vi "ReadEyeFileFast.vi"(0 "new file path":path=path "C:/WINDOWS/DESKTOP/rri.eye", 6 "Header format":u16(ring) items=["Riverside Format", "Ron Linear", "GE Bin"]) -> (8 "Complex output array":csg[][](array[numeric]), 9 "Digitizer (dB)":sgl, 10 "new path out":path, 11 "RF Att":sgl format="%.2f", 13 "2-D data array":sgl[][](array[numeric]), 14 "Header In":T1={"header info"={"Header"="", "Head length"=0}, "A/D info"={"# rf points per line"=0, "# lines per scan"=0, "sample rate MHz"=0, "# A/D bits"=0, "# bytes per A/D"=0, "TGC Flag"=0, "A/D Type"=""}, "Tranducer Info"={"bandwidth"=0.0, "center freq"=0.0, "start freq"=0.0, "ID"=0}, "Scan Info"={"delay"=0.0, "pivot distance"=0.0, "sector scan angle"=0.0, "operator"="", "Scan Mode"="", "location"=""}, "Time/Date Info"={"date"="", "time"=""}, "RF Info"={"RF file name"="", "RF file att"="", "RF cal file name"="", "RF cal file att"=""}, "Patient Info"={"ID"="", "extended ID"="", "age"=0, "sex"="", "previously\nscanned"="", "PSA"=0.0, "LOS"=1, "Ethnicty 2"=3, "Race"=3}, "Tissue Type"={"organ"=0, "disease type"=0, "disease location"=0, "IQ_pts"=0, "RcvBuffer"=0, "RcvFrame"=0, "IQBuff"=0, "IQFrame"=0, "IQPage"=0}, "Votage scaling"={"Digitizer (dB)"=0.0, "Gain (dB)"=0.0, "Atten (dB)"=0.0}, "Comment"="", "Misc Info"={"avg num"=0, "c speed"=0, "Div By or SF zones"=0, "XMIT CHS"=0, "RCV CHS"=0, "Xmit angle"=0.0}, "Therapy Parameters"={"Theraputic Freq (MHz)"=0.0, "Time on (s)"=0.0, "Therapy amplitude (mV)"=0.0, "Lines Before"=0, "Lines After"=0}, "Scan Settings"={"Energy (uJ or V)"=0, "Damp (Ohm) or Fc"=0, "HP Filt (KHz)"=0, "LP Filt (MHz)"=0, "Gain (db)"=0, "prf (kHz)"=0.0, "Distance between\nscan lines (um)"=0, "Distance between\nscan planes (um)"=0, "Scan line gap (um)"=0.0, "Scan plane gap (um)"=0.0}, "Compression Parameters"={"F1 (MHz)"=0.0, "F2 (MHz)"=0.0, "% taper"=0.0, "duration"=0.0}, "Patient Info Xtra"={"First Name"="", "Last Name"="", "Notes"=""}, "ROI Box"=[0, 0, 0, 0]} {"Compression Parameters"."% taper" min=50 max=1000 format="%.2f"; "Compression Parameters"."F2 (MHz)" format="%.3f"; "Compression Parameters"."F1 (MHz)" format="%.3f"; "Scan Settings"."prf (kHz)" format="%.2f"; "Therapy Parameters"."Therapy amplitude (mV)" min=50 max=1000 format="%.2f"; "Therapy Parameters"."Time on (s)" format="%.3f"; "Therapy Parameters"."Theraputic Freq (MHz)" format="%.3f"; "Patient Info"."Race" items=["Am Ind or Alaska", "Asian", "Hawaiian, Pac Isl", "Black or Afr Amer", "White", "more than one race", "unknown"]; "Patient Info"."Ethnicty 2" items=["Hispanic", "Non-Hispanic", "unknown"]; "Patient Info"."LOS" items=["1", "2", "3", "4", "5"]; "Patient Info"."PSA" format="%.1f"; "Scan Info"."delay" format="%.2f"; "Scan Info"."pivot distance" format="%.2f"; "Scan Info"."sector scan angle" format="%.2f"; "Tranducer Info"."bandwidth" format="%.2f"; "Tranducer Info"."center freq" format="%.2f"; "Tranducer Info"."start freq" format="%.2f"})   [LabVIEW 2022 SP3]
uses:
  Header.ctl
panel:
  out "error out":errorcluster
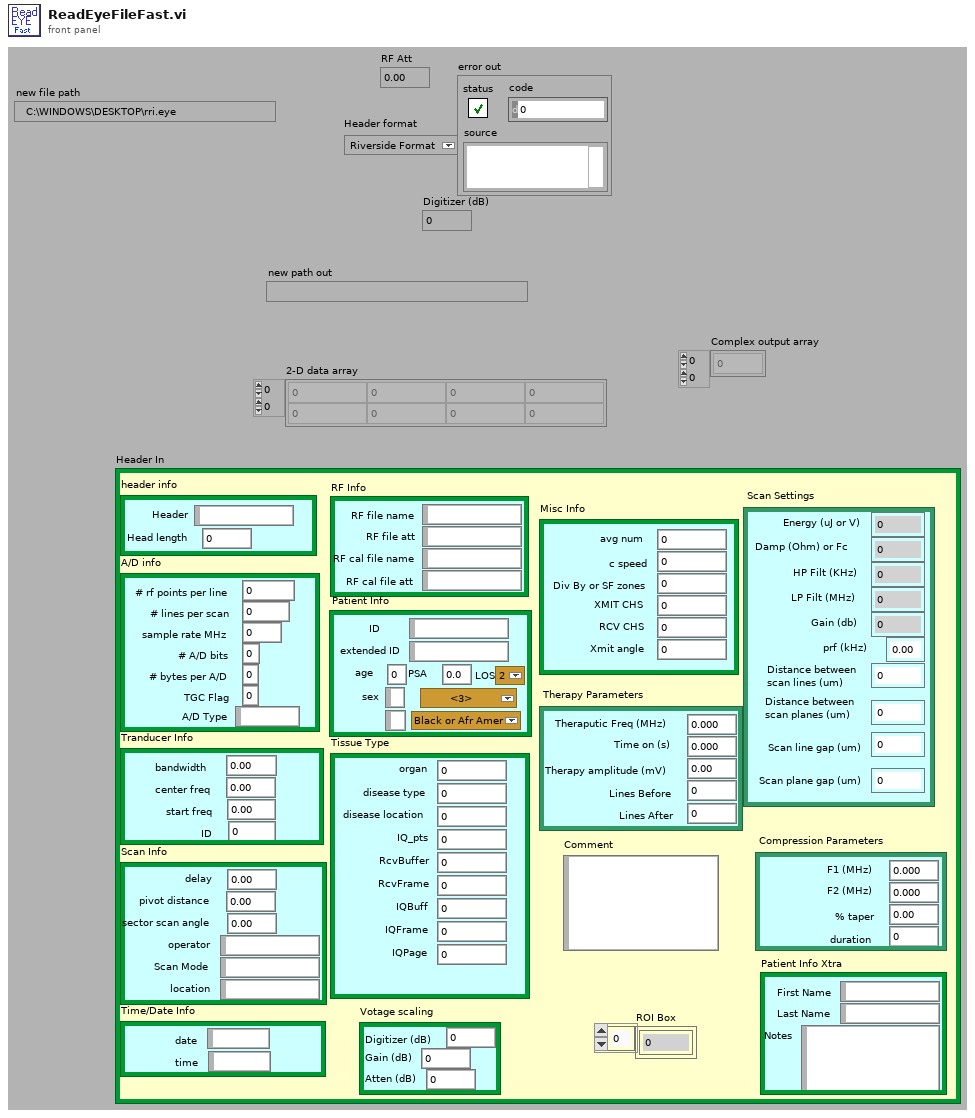
[diagram p1: front panel]
types:
  T1 = typedef "Header.ctl" = cluster{"header info":cluster{"Header":string, "Head length":i16}, "A/D info":cluster{"# rf points per line":u16, "# lines per scan":u16, "sample rate MHz":u16, "# A/D bits":i16, "# bytes per A/D":u16, "TGC Flag":u16, "A/D Type":string}, "Tranducer Info":cluster{"bandwidth":sgl, "center freq":sgl, "start freq":sgl, "ID":i32}, "Scan Info":cluster{"delay":sgl, "pivot distance":sgl, "sector scan angle":sgl, "operator":string, "Scan Mode":string, "location":string}, "Time/Date Info":cluster{"date":string, "time":string}, "RF Info":cluster{"RF file name":string, "RF file att":string, "RF cal file name":string, "RF cal file att":string}, "Patient Info":cluster{"ID":string, "extended ID":string, "age":u16, "sex":string, "previously\nscanned":string, "PSA":sgl, "LOS":u8, "Ethnicty 2":u8, "Race":u8}, "Tissue Type":cluster{"organ":i16, "disease type":i16, "disease location":i16, "IQ_pts":u16, "RcvBuffer":u8, "RcvFrame":u16, "IQBuff":u8, "IQFrame":u16, "IQPage":u8}, "Votage scaling":cluster{"Digitizer (dB)":sgl, "Gain (dB)":sgl, "Atten (dB)":sgl}, "Comment":string, "Misc Info":cluster{"avg num":u16, "c speed":i16, "Div By or SF zones":i16, "XMIT CHS":u8, "RCV CHS":u8, "Xmit angle":sgl}, "Therapy Parameters":cluster{"Theraputic Freq (MHz)":sgl, "Time on (s)":sgl, "Therapy amplitude (mV)":sgl, "Lines Before":u16, "Lines After":u16}, "Scan Settings":cluster{"Energy (uJ or V)":u8, "Damp (Ohm) or Fc":u8, "HP Filt (KHz)":u8, "LP Filt (MHz)":u8, "Gain (db)":u8, "prf (kHz)":sgl, "Distance between\nscan lines (um)":u16, "Distance between\nscan planes (um)":u16, "Scan line gap (um)":sgl, "Scan plane gap (um)":sgl}, "Compression Parameters":cluster{"F1 (MHz)":sgl, "F2 (MHz)":sgl, "% taper":sgl, "duration":sgl}, "Patient Info Xtra":cluster{"First Name":string, "Last Name":string, "Notes":string}, "ROI Box":u16[]}
  T2 = enum16{"big-endian, network order", "native, host order", "little-endian"}
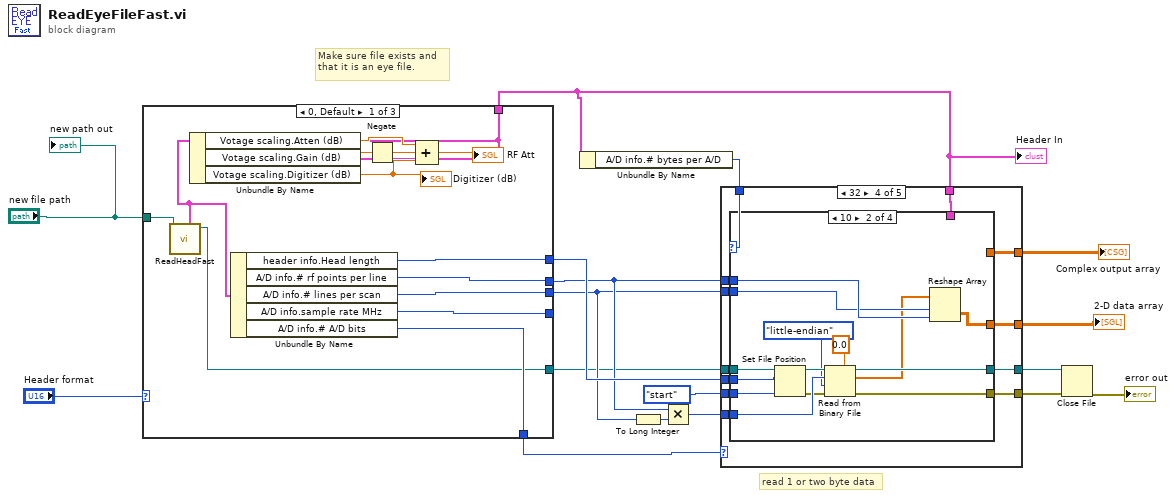
[diagram p0: block diagram]
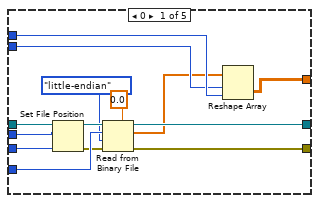
[diagram p2: hidden frame]
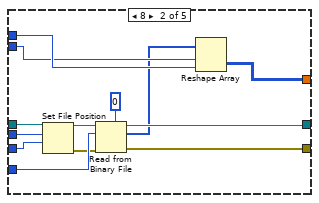
[diagram p3: hidden frame]
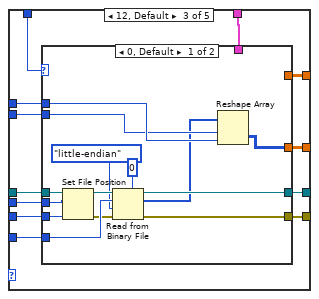
[diagram p4: hidden frame]
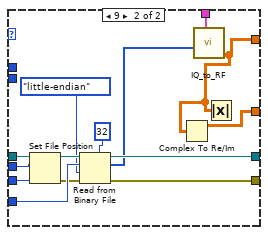
[diagram p5: hidden frame]
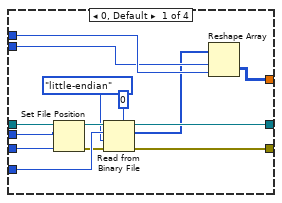
[diagram p6: hidden frame]
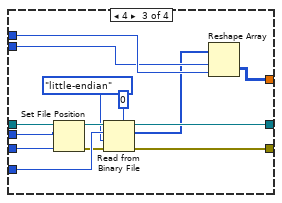
[diagram p7: hidden frame]
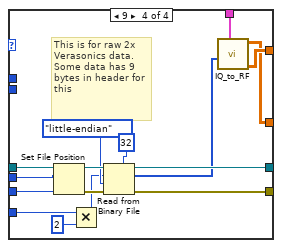
[diagram p8: hidden frame]
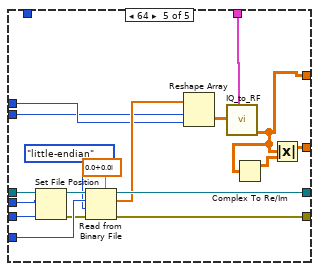
[diagram p9: hidden frame]
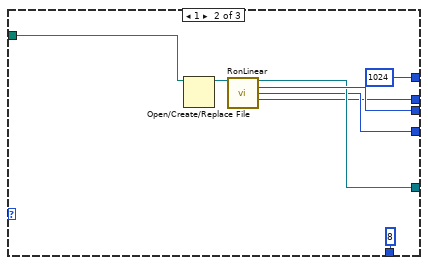
[diagram p10: hidden frame]
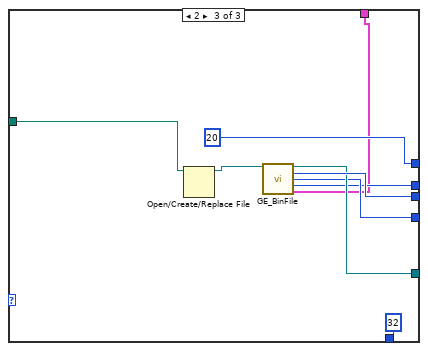
[diagram p11: hidden frame]
diagram:
  # "Make sure file exists and that it is an eye file."
  # "read 1 or two byte data"
  n1 = case shown="0, Default" "Header format" {
    tunnel: [w26 w35 w44] -> _
    tunnel: [w28 w33 w42] -> w7
    tunnel: [w27 w38 w47] -> w6
    tunnel: [w19 w37 w46] -> w2
    tunnel: [w29 i16 1024 i16 20] -> w12
    tunnel: [w25 8 32] -> w8
    tunnel: "new file path" -> [w30 w31 w40]
    tunnel: [w18 _ w39] -> w4
    frame 0, Default {
      n2 = call "ReadHeadFast.vi"("new file path"=w30) -> ("refnum out"=w19:refnum<file>, "Header In"=w18:T1)  [unwired: 7 in, 2 out]
      n3 = Unbundle By Name(w18) -> ("Votage scaling.Atten (dB)"=w20:sgl, "Votage scaling.Gain (dB)"=w23:sgl, "Votage scaling.Digitizer (dB)"=w24:sgl)
      "Digitizer (dB)" <- w24
      n4 = Unbundle By Name(w18) -> ("header info.Head length"=w29:i16, "A/D info.# rf points per line"=w28:u16, "A/D info.# lines per scan"=w27:u16, "A/D info.sample rate MHz"=w26:u16, "A/D info.# A/D bits"=w25:i16)
      n5 = Negate(x=w23) -> (-x=w21:sgl)
      n6 = Compound Arithmetic op=ADD(w20, w21, w24) -> (→"RF Att":sgl)
    }
    frame 1 {
      n7 = Open/Create/Replace File(file path (use dialog)=w31) -> (refnum out=w32:refnum<file>)  [unwired: 5 in, 2 out]
      n8 = call "RonLinear.vi"("refnum"=w32) -> ("refnum out"=w37:refnum<file>, "# lines per scan"=w38:i32, "sample rate"=w35:u16, "# rf points per line"=w33:u16)  [unwired: 11 out]
    }
    frame 2 {
      n9 = Open/Create/Replace File(file path (use dialog)=w40) -> (refnum out=w41:refnum<file>)  [unwired: 5 in, 2 out]
      n10 = call "GE_BinFile.vi"("refnum"=w41) -> ("refnum out"=w46:refnum<file>, "# lines per scan"=w47:i32, "sample rate"=w44:u16, "# rf points per line"=w42:u16, "Header In"=w39:T1)  [unwired: 9 in, 1 out]
    }
  }
  "Header In" <- w4
  n11 = Unbundle By Name(w4) -> ("A/D info.# bytes per A/D"=w5:u16)
  n12 = To Long Integer(number=w6) -> (32bit integer=w15:i32)
  n13 = Multiply(x=w7, y=w15) -> (x*y=w16:i32)
  n14 = case shown="32" w8 {
    tunnel: enum16{"start", "end", "current"}."start" ("pos mode (0:2)") -> [w58 w73 w84 w124 w198]
    tunnel: [w48 w62 w78 w118 w185] -> w3
    tunnel: w16 -> [w59 w72 w85 w125 w199]
    tunnel: w2 -> [w61 w71 w86 w126 w201]
    tunnel: w12 -> [w54 w70 w82 w122 w194]
    tunnel: [w57 w69 w83 w123 w197] -> w13
    tunnel: [w52 w66 w81 w121 w192] -> w11
    tunnel: w7 -> [w51 w65 w80 w120 w190]
    tunnel: w6 -> [w50 w64 w79 w119 w189]
    tunnel: w4 -> [_ _ w76 w116 w188]
    tunnel: w5 -> [_ _ w77 w117 _]
    tunnel: [_ _ w75 w115 w186] -> w1
    frame 0 {
      n15 = Set File Position(offset (in bytes) (0)=w54, refnum=w61, from (0:start)=w58) -> (refnum out=w56:refnum<file>, error out=w55:errorcluster)  [unwired: 1 in]
      n16 = Read from Binary File(5:sgl 0.0, 8:w55, 9:T2."little-endian" ("byte order (0:big-endian, network order)"), 10:w59, 11:w56) -> (0:w52:errorcluster, 2:w49:sgl[], 3:w57:refnum<file>)  [unwired: 2 out]
      n17 = Reshape Array(w49, w50, w51) -> (w48:sgl[][])
    }
    frame 8 {
      n18 = Set File Position(offset (in bytes) (0)=w70, refnum=w71, from (0:start)=w73) -> (refnum out=w68:refnum<file>, error out=w67:errorcluster)  [unwired: 1 in]
      n19 = Read from Binary File(5:i8 0, 8:w67, 10:w72, 11:w68) -> (0:w66:errorcluster, 2:w63:i8[], 3:w69:refnum<file>)  [unwired: 3 out]
      n20 = Reshape Array(w63, w64, w65) -> (w62:i8[][])
    }
    frame 12, Default {
      n21 = case shown="0, Default" w77 {
        tunnel: w86 -> [w100 w114]
        tunnel: w85 -> [w98 w112]
        tunnel: w84 -> [w97 w111]
        tunnel: [w96 w110] -> w83
        tunnel: w82 -> [w93 w107]
        tunnel: [w91 w105] -> w81
        tunnel: w80 -> [w90 _]
        tunnel: w79 -> [w89 _]
        tunnel: [w87 w101] -> w78
        tunnel: w76 -> [_ w104]
        tunnel: [_ w102] -> w75
        frame 0, Default {
          n22 = Set File Position(offset (in bytes) (0)=w93, refnum=w100, from (0:start)=w97) -> (refnum out=w95:refnum<file>, error out=w94:errorcluster)  [unwired: 1 in]
          n23 = Read from Binary File(5:i16 0, 8:w94, 9:T2."little-endian" ("byte order (0:big-endian, network order)"), 10:w98, 11:w95) -> (0:w91:errorcluster, 2:w88:i16[], 3:w96:refnum<file>)  [unwired: 2 out]
          n24 = Reshape Array(w88, w89, w90) -> (w87:i16[][])
        }
        frame 9 {
          n25 = Set File Position(offset (in bytes) (0)=w107, refnum=w114, from (0:start)=w111) -> (refnum out=w109:refnum<file>, error out=w108:errorcluster)  [unwired: 1 in]
          n26 = Read from Binary File(5:32, 8:w108, 9:T2."little-endian" ("byte order (0:big-endian, network order)"), 10:w112, 11:w109) -> (0:w105:errorcluster, 2:w103:i32[], 3:w110:refnum<file>)  [unwired: 2 out]
          n27 = call "IQ_to_RF.vi"("Header In"=w104, "IQ Array In"=w103) -> ("Z Out"=w102:csg[][])  [unwired: 8 in, 1 out]
          n28 = Complex To Re/Im(x + iy=w102) -> (x=w101:sgl[][])  [unwired: 1 out]
          n29 = Absolute Value(x=w102) -> ()  [unwired: 1 out]
        }
      }
    }
    frame 32 {
      n30 = case shown="10" w117 {
        tunnel: w126 -> [w140 w154 w168 w184]
        tunnel: w125 -> [w138 w152 w166 w173]
        tunnel: w124 -> [w137 w151 w165 w182]
        tunnel: [w136 w150 w164 w181] -> w123
        tunnel: w122 -> [w133 w147 w161 w178]
        tunnel: [w131 w145 w159 w176] -> w121
        tunnel: w120 -> [w130 w144 w158 _]
        tunnel: w119 -> [w129 w143 w157 _]
        tunnel: [w127 w141 w155 w169] -> w118
        tunnel: w116 -> [_ _ _ w175]
        tunnel: [_ _ _ w170] -> w115
        frame 0, Default {
          n31 = Set File Position(offset (in bytes) (0)=w133, refnum=w140, from (0:start)=w137) -> (refnum out=w135:refnum<file>, error out=w134:errorcluster)  [unwired: 1 in]
          n32 = Read from Binary File(5:0, 8:w134, 9:T2."little-endian" ("byte order (0:big-endian, network order)"), 10:w138, 11:w135) -> (0:w131:errorcluster, 2:w128:i32[], 3:w136:refnum<file>)  [unwired: 2 out]
          n33 = Reshape Array(w128, w129, w130) -> (w127:i32[][])
        }
        frame 10 {
          n34 = Set File Position(offset (in bytes) (0)=w147, refnum=w154, from (0:start)=w151) -> (refnum out=w149:refnum<file>, error out=w148:errorcluster)  [unwired: 1 in]
          n35 = Read from Binary File(5:sgl 0.0, 8:w148, 9:T2."little-endian" ("byte order (0:big-endian, network order)"), 10:w152, 11:w149) -> (0:w145:errorcluster, 2:w142:sgl[], 3:w150:refnum<file>)  [unwired: 2 out]
          n36 = Reshape Array(w142, w143, w144) -> (w141:sgl[][])
        }
        frame 4 {
          n37 = Set File Position(offset (in bytes) (0)=w161, refnum=w168, from (0:start)=w165) -> (refnum out=w163:refnum<file>, error out=w162:errorcluster)  [unwired: 1 in]
          n38 = Read from Binary File(5:0, 8:w162, 9:T2."little-endian" ("byte order (0:big-endian, network order)"), 10:w166, 11:w163) -> (0:w159:errorcluster, 2:w156:i32[], 3:w164:refnum<file>)  [unwired: 2 out]
          n39 = Reshape Array(w156, w157, w158) -> (w155:i32[][])
        }
        frame 9 {
          # "This is for raw 2x\nVerasonics data.\nSome data has 9 bytes in header for this"
          n40 = Set File Position(offset (in bytes) (0)=w178, refnum=w184, from (0:start)=w182) -> (refnum out=w180:refnum<file>, error out=w179:errorcluster)  [unwired: 1 in]
          n41 = Multiply(x=w173, y=2) -> (x*y=w172:i32)
          n42 = Read from Binary File(5:32, 8:w179, 9:T2."little-endian" ("byte order (0:big-endian, network order)"), 10:w172, 11:w180) -> (0:w176:errorcluster, 2:w174:i32[], 3:w181:refnum<file>)  [unwired: 2 out]
          n43 = call "IQ_to_RF.vi"("Header In"=w175, "IQ Array In"=w174) -> ("Z Out"=w170:csg[][], "RF Array"=w169:sgl[][])  [unwired: 8 in]
        }
      }
    }
    frame 64 {
      n44 = Set File Position(offset (in bytes) (0)=w194, refnum=w201, from (0:start)=w198) -> (refnum out=w196:refnum<file>, error out=w195:errorcluster)  [unwired: 1 in]
      n45 = Read from Binary File(5:csg 0.0+0.0i, 8:w195, 9:T2."little-endian" ("byte order (0:big-endian, network order)"), 10:w199, 11:w196) -> (0:w192:errorcluster, 2:w191:csg[], 3:w197:refnum<file>)  [unwired: 2 out]
      n46 = Reshape Array(w191, w189, w190) -> (w187:csg[][])
      n47 = call "IQ_to_RF.vi"("Header In"=w188, "IQ Array"=w187) -> ("Z Out"=w186:csg[][])  [unwired: 8 in, 1 out]
      n48 = Complex To Re/Im(x + iy=w186) -> (x=w185:sgl[][])  [unwired: 1 out]
      n49 = Absolute Value(x=w186) -> ()  [unwired: 1 out]
    }
  }
  "2-D data array" <- w3
  "Complex output array" <- w1
  n50 = Close File(refnum=w13, error in=w11) -> (error out=→"error out":errorcluster)  [unwired: 1 out]
  "new path out" <- "new file path"
